vi "Table, Get Cell Color.vi"(8 "error in":errorcluster, 9 "col (0)":i32, 10 "row (0)":i32, 11 "Tbl Refnum":refnum<vi>) -> (0 "error out":errorcluster, 1 "col+1":i32, 2 "row+1":i32, 3 "Tbl Refnum out":refnum<vi>, 5 "BGColor":u32(colorbox)=16744640)   [LabVIEW 2010]
doc: "This function sets the active table cell and gets its background color attribute."
uses:
  <vilib>/Utility/miscctls.llb/LVRowAndColumnTypeDef.ctl
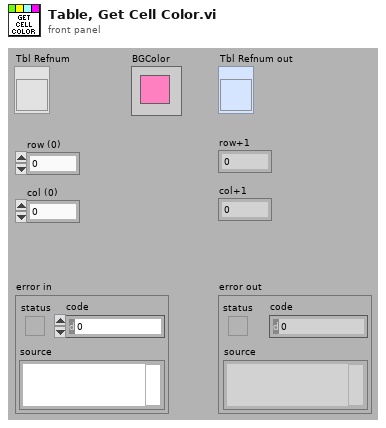
[diagram p1: front panel]
types:
  T1 = typedef "LVRowAndColumnTypeDef.ctl" = cluster{"Row":i32, "Column":i32}
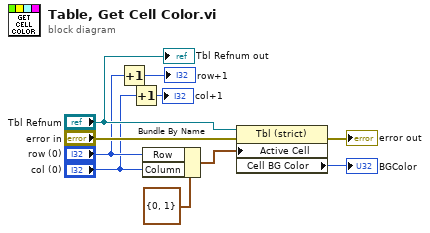
[diagram p0: block diagram]
diagram:
  n1 = Increment(x="row (0)") -> (x+1=→"row+1":i32)
  n2 = Increment(x="col (0)") -> (x+1=→"col+1":i32)
  n3 = Bundle By Name(cluster=T1 {"Row"=0, "Column"=1} ("Selection Start 2"), "Row"="row (0)", "Column"="col (0)") -> (w7:T1)
  n4 = property class="Tbl (strict)"(reference="Tbl Refnum", error in="error in", "Active Cell"=w7) -> (error out=→"error out":errorcluster, "Cell BG Color"=→"BGColor":u32)  [unwired: 1 out]
  "Tbl Refnum out" <- "Tbl Refnum"
